vi "sensor get device id list.vi"(10 "buffer_length":u32, 11 "serial_number_buffer":u32) -> (2 "function return":i32, 3 "serial_number_buffer out":u32)   [LabVIEW 2019, in "apdm.lvlib"]
doc: "APDM_DEPRECATED APDM_EXPORT int apdm_sensor_get_device_id_list(uint32_t *serial_number_buffer, const uint32_t buffer_length);"
uses:
  apdm.lvlib
  Lee Lab/CP FES Walking 2018/Code/Working/LabVIEW/apdm.dll
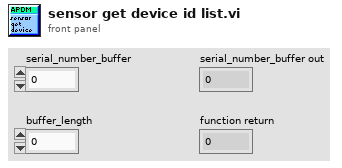
[diagram p1: front panel]
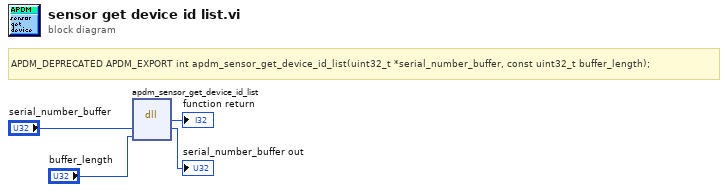
[diagram p0: block diagram]
diagram:
  # "APDM_DEPRECATED APDM_EXPORT int apdm_sensor_get_device_id_list(uint32_t *serial_number_buffer, const uint32_t buffer_length);"
  n1 = dll-call lib="C:/Users/jfalesi/Dropbox/Lee Lab/CP FES Walking 2018/Code/Working/LabVIEW/apdm.*" fn="apdm_sensor_get_device_id_list"("serial_number_buffer"="serial_number_buffer", "buffer_length"="buffer_length") -> (→"function return":i32, "serial_number_buffer"=→"serial_number_buffer out":u32)  [unwired: 4 in, 2 out]
